vi "Instrument.sendMessageToProcess.vi"   [LabVIEW 2019, in "Instrument.lvlib" / "Instrument.lvclass"]
doc: "Send a message (<b>Command</b>, <b>Data</b>, <b>ID</b>) <b>to</b> Instrument.lvclass:process.vi\n\nThis polymorphic VI supports two datatypes for <b>Command</b>: <b>string</b> or <b>variant</b> (where <b>variant</b> is really an <b>enum</b>)"
uses:
  Instrument.lvclass
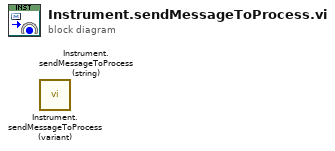
[diagram p0: block diagram]
diagram:
  n1 = call "Instrument.sendMessageToProcess (variant).vi"() -> ()  [unwired: 10 in, 2 out]
  n2 = call "Instrument.sendMessageToProcess (string).vi"() -> ()  [unwired: 10 in, 2 out]
